vi "SwerveDriveLogic.vi"(9 "Speeds":dbl[](array[numeric]), 10 "AngleSetpoints":dbl[](array[numeric]), 11 "AngleEncoders":dbl[](array[numeric])) -> (2 "AngleMotorsReversed":bool[](array[boolean]), 3 "AngleMotorOutputs":dbl[](array[numeric]))   [LabVIEW 2017]
uses:
  <vilib>/addons/control/pid/pid.llb/PID (DBL).vi
  <vilib>/addons/control/pid/NI_PID_pid.lvlib
panel:
  in  "PID gains":T1={"proportional gain (Kc)"=0.025, "integral time (Ti, min)"=0.003, "derivative time (Td, min)"=0.0} {"derivative time (Td, min)" format="%.3f"; "integral time (Ti, min)" format="%.3f"; "proportional gain (Kc)" format="%.3f"}
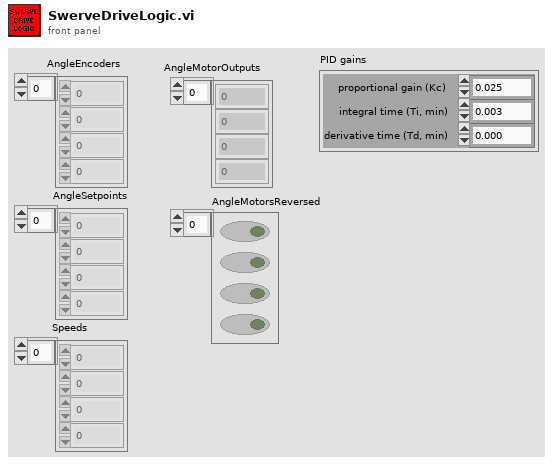
[diagram p1: front panel]
types:
  T1 = cluster{"proportional gain (Kc)":dbl, "integral time (Ti, min)":dbl, "derivative time (Td, min)":dbl}
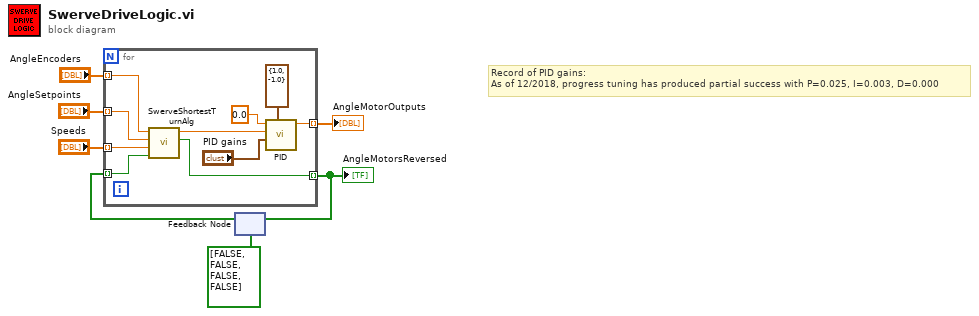
[diagram p0: block diagram]
diagram:
  # "Record of PID gains:\nAs of 12/2018, progress tuning has produced partial success with P=0.025, I=0.003, D=0.000"
  n1 = feedback #1(bool[] [FALSE, FALSE, FALSE, FALSE] ("SwerveMotorsFlipped")) -> (w6:bool[])
  n2 = for {
    tunnel: "AngleEncoders" -> [w9] mode=indexing
    tunnel: "Speeds" -> [w15] mode=indexing
    tunnel: w6 -> [w11] mode=indexing
    tunnel: "AngleSetpoints" -> [w10] mode=indexing
    tunnel: [w14] -> w3 mode=indexing
    tunnel: [w13] -> w5 mode=indexing
    n3 = call "SwerveShortestTurnAlg.vi"("SwerveMotorsFlipped?"=w11, "SwerveSpeed"=w15, "AngleSetpoint"=w10, "AngleEncoder"=w9) -> ("FlipSwerveMotors"=w13:bool, "PIDInput"=w8:dbl)  [unwired: 6 in]
    n4 = call-poly <vilib>:"PID.vi"("output range"=cluster{"output high":dbl, "output low":dbl} {"output high"=1.0, "output low"=-1.0}, "PID gains"="PID gains", "process variable"=w8, "setpoint"=0.0) -> ("output"=w14:dbl)  [unwired: 6 in, 1 out]
  }
  "AngleMotorOutputs" <- w3
  "AngleMotorsReversed" <- w5
  n5 = feedback-in #1(w5) -> ()
